vi "Proceed.vi"(7 "component is ready (Y)":bool=TRUE, 8 "error in (no error)":errorcluster, 10 "ProceedMessage":refnum<class "ProceedMessage.lvclass">, 11 "Cascade in":refnum<class "Cascade.lvclass">) -> (0 "error out":errorcluster, 2 "all observers are ready?":bool, 3 "Cascade out":refnum<class "Cascade.lvclass">)   [LabVIEW 2012, in "Cascade.lvclass"]
doc: "The Proceed method is used to check if your component is ready. Also it checks if the observers are ready. When the observers and the component are ready, it sends the proceed to its observee. If it's the highest observee, it distributes a stop command."
uses:
  Cascade.lvclass
  <vilib>/Distrio/Murmex/ProceedMessage/ProceedMessage.lvclass
  Cascade.lvclass/Cascade.ctl
  <vilib>/Distrio/Murmex/GenericMessage/GenericMessage.lvclass
  <vilib>/Distrio/Murmex/Murmex/Murmex.lvclass
  <vilib>/Distrio/Murmex/Message/Add or replace parameter.vi
  <vilib>/Distrio/Murmex/Message/Message.lvclass
panel:
  # "This method is called when the PROCEED\ntrigger is sent. \n\nOverride this method when your component needs to\nrespond to this trigger. \n\nCall parent for proper implementation"
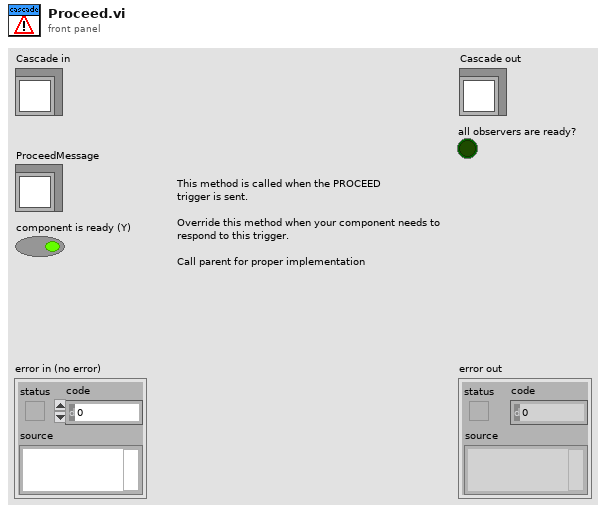
[diagram p1: front panel]
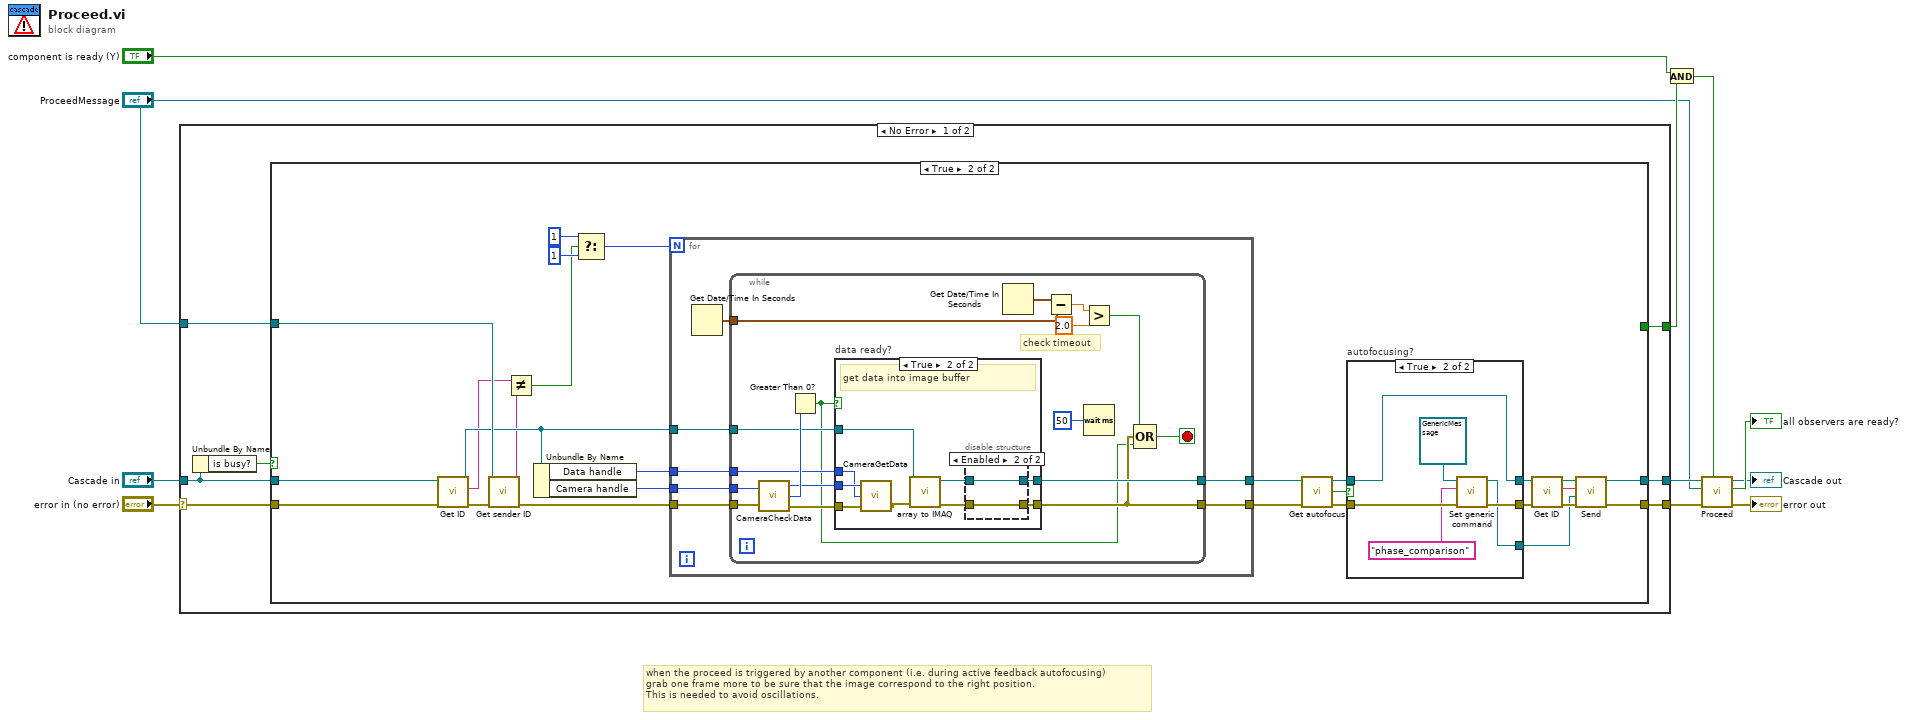
[diagram p0: block diagram]
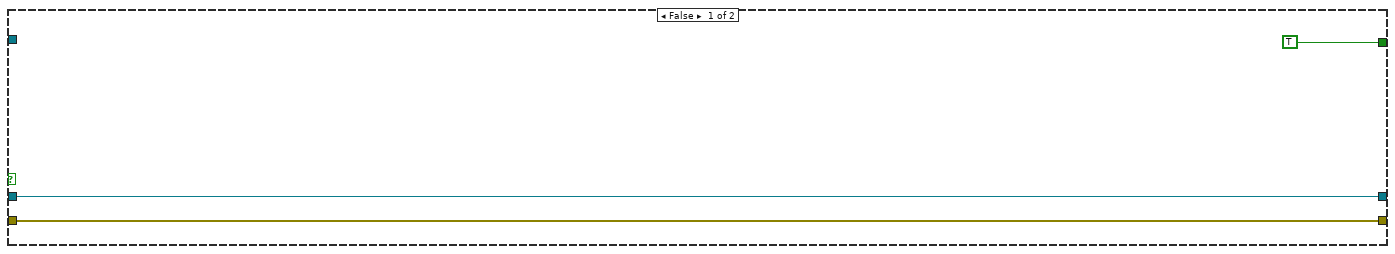
[diagram p2: hidden frame]
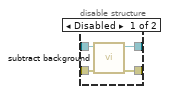
[diagram p4: hidden frame]
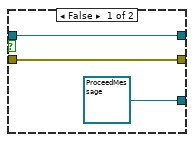
[diagram p5: hidden frame]
diagram:
  # "when the proceed is triggered by another component (i.e. during active feedback autofocusing)\ngrab one frame more to be sure that the image correspond to the right position.\nThis is needed to avoid oscillations."
  n1 = case shown="No Error" "error in (no error)" {
    selector: "error in (no error)" -> [w18 w100]
    tunnel: "Cascade in" -> [w17 w99]
    tunnel: [w15 w100] -> w7
    tunnel: [w14 w99] -> w6
    tunnel: [w13 _] -> w4
    tunnel: "ProceedMessage" -> [w12 _]
    frame No Error {
      n2 = Unbundle By Name(w17) -> ("is busy?"=w16:bool)
      n3 = case shown="True" w16 {
        tunnel: w18 -> [w20 w48]
        tunnel: w17 -> [w19 w47]
        tunnel: [w20 w46] -> w15
        tunnel: [w19 w45] -> w14
        tunnel: [TRUE _] -> w13
        tunnel: w12 -> [_ w44]
        frame False {
        }
        frame True {
          n4 = call <vilib>:"Get ID.vi"("error in (no error)"=w48, "Murmex in"=w47) -> ("error out"=w29:errorcluster, "component id"=w27:string, "Murmex out"=w30:refnum<class "Cascade.lvclass">)  [unwired: 7 in]
          n5 = call <vilib>:"Get sender ID.vi"("error in (no error)"=w29, "Message in"=w44) -> ("error out"=w28:errorcluster, "sender"=w26:string)  [unwired: 7 in, 1 out]
          n6 = Not Equal?(x=w27, y=w26) -> (x != y?=w23:bool)
          n7 = Unbundle By Name(w30) -> ("Data handle"=w42:u32, "Camera handle"=w43:u32)
          n8 = Select(t=1, s=w23, f=1) -> (s? t:f=w22:i32)
          n9 = for {
            N: w22 -> [_]
            tunnel: w43 -> [w55]
            tunnel: w42 -> [w54]
            tunnel: [w53] -> w41
            tunnel: [w52] -> w36
            tunnel: w30 -> [w50]
            tunnel: w28 -> [w49]
            n10 = Get Date/Time In Seconds() -> (seconds since 1Jan1904=w51:timestamp)
            n11 = while {
              tunnel: w49 -> [w69]
              tunnel: [w58] -> w53
              tunnel: w55 -> [w68]
              tunnel: w54 -> [w67]
              tunnel: w50 -> [w66]
              tunnel: [w65] -> w52
              tunnel: w51 -> [w62]
              stop <- w56 stop-if-true
              # "check timeout"
              n12 = call <userlib>:"CameraCheckData.vi"("Camera Handle"=w68, "error in"=w69) -> ("Camera Handle"=w70:u32, "Number Of Frames Available"=w71:i32, "error out"=w72:errorcluster)
              n13 = Greater Than 0?(x=w71) -> (x > 0?=w57:bool)
              n14 = case "data ready?" shown="True" w57 {
                tunnel: w72 -> [w74 w83]
                tunnel: w70 -> [_ w82]
                tunnel: [w74 w77] -> w58
                tunnel: w67 -> [_ w81]
                tunnel: w66 -> [w73 w80]
                tunnel: [w73 w75] -> w65
                frame False {
                }
                frame True {
                  # "get data into image buffer"
                  n15 = call <userlib>:"CameraGetData.vi"("error in"=w83, "Data Handle"=w81, "Camera Handle"=w82) -> ("error out"=w79:errorcluster)  [unwired: 2 out]
                  n16 = call-dynamic "array to IMAQ.vi"("error in (no error)"=w79, "Cascade in"=w80) -> ("error out"=w78:errorcluster, "Cascade out"=w76:refnum<class "Cascade.lvclass">)  [unwired: 8 in]
                  n17 = disable-structure shown="Enabled" {
                    disable-tunnel: w78 -> [w87 w88]
                    disable-tunnel: [w86 w88] -> w77
                    disable-tunnel: w76 -> [w85 w89]
                    disable-tunnel: [w84 w89] -> w75
                    frame Disabled {
                      n18 = call-dynamic "subtract background.vi"("error in (no error)"=w87, "Cascade in"=w85) -> ("error out"=w86:errorcluster, "Cascade out"=w84:refnum<class "Cascade.lvclass">)  [unwired: 8 in]
                    }
                    frame Enabled {
                    }
                  }
                }
              }
              n19 = Get Date/Time In Seconds() -> (seconds since 1Jan1904=w63:timestamp)
              n20 = Subtract(x=w63, y=w62) -> (x-y=w61:dbl)
              n21 = Greater?(x=w61, y=2.0) -> (0:w59:bool)
              n22 = Wait (ms)(milliseconds to wait=u32 50) -> ()  [unwired: 1 out]
              n23 = Compound Arithmetic op=OR(w59, w58, w57) -> (w56:bool)
            }
          }
          n24 = call-dynamic "Get autofocus.vi"("error in (no error)"=w41, "Cascade in"=w36) -> ("error out"=w33:errorcluster, "autofocusing?"=w35:bool, "Cascade out"=w32:refnum<class "Cascade.lvclass">)  [unwired: 7 in]
          n25 = case "autofocusing?" shown="True" w35 {
            tunnel: [refnum<class "ProceedMessage.lvclass"> refnum ("Distrio Murmex 1.5:ProceedMessage") w96] -> w38
            tunnel: [w91 w97] -> w34
            tunnel: w33 -> [w91 w98]
            tunnel: w32 -> [w90 w95]
            tunnel: [w90 w95] -> w31
            frame False {
            }
            frame True {
              n26 = call <vilib>:"Set generic command.vi"("error in (no error)"=w98, "generic command"="phase_comparison", "GenericMessage in"=refnum<class "GenericMessage.lvclass"> refnum ("Message in")) -> ("error out"=w97:errorcluster, "GenericMessage out"=w96:refnum<class "GenericMessage.lvclass">)  [unwired: 7 in]
            }
          }
          n27 = call <vilib>:"Get ID.vi"("error in (no error)"=w34, "Murmex in"=w31) -> ("error out"=w40:errorcluster, "component id"=w37:string, "Murmex out"=w39:refnum<class "Cascade.lvclass">)  [unwired: 7 in]
          n28 = call <vilib>:"Send.vi"("error in (no error)"=w40, "Message"=w38, "recipient"=w37, "Murmex in"=w39) -> ("error out"=w46:errorcluster, "Murmex out"=w45:refnum<class "Cascade.lvclass">)  [unwired: 6 in]
        }
      }
    }
    frame Error {
    }
  }
  n29 = And(x="component is ready (Y)", y=w4) -> (x .and. y?=w2:bool)
  n30 = call-parent "Proceed.vi"("component is ready (Y)"=w2, "error in (no error)"=w7, "ProceedMessage"="ProceedMessage", "Murmex in"=w6) -> ("error out"=→"error out":errorcluster, "all observers are ready?"=→"all observers are ready?":bool, "Murmex out"=→"Cascade out":refnum<class "Cascade.lvclass">)  [unwired: 5 in]
